vi "test.vi"() -> ()   [LabVIEW 2014]
uses:
  <vilib>/Utility/miscctls.llb/LVRectTypeDef.ctl
  <vilib>/Analysis/NI_AALBase.lvlib
panel:
  out "Numeric":i32
  out "Histogram Graph":T1(graph)
  in  "intervals":i32=10
  out "x-y":u32
  out "Image 2":u8[][](graph) caption="Image"
  out "framerate":dbl
  out "exposure":dbl
  in  "Exposure[ms]":dbl=100.0 format="%#_13g"
  out "SizeOut":T2
  in  "SizeIn":T2={"posX"=0, "posY"=0, "Width"=1024, "height"=1024}
  in  "stop":bool
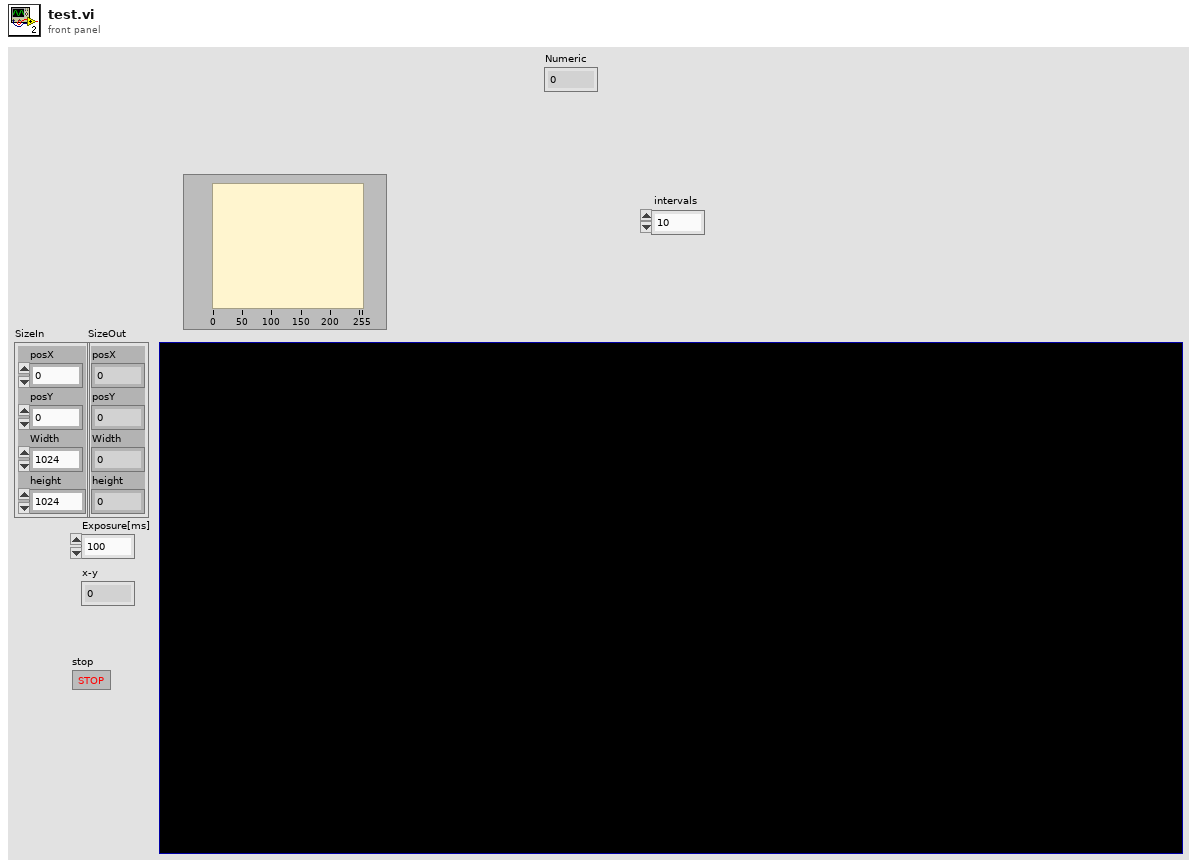
[diagram p1: front panel]
types:
  T1 = cluster{"X Values":dbl[], "Histogram: h(x)":i32[]}
  T2 = cluster{"posX":i32, "posY":i32, "Width":i32, "height":i32}
  T3 = typedef "LVRectTypeDef.ctl" = cluster{"Left":i16, "Top":i16, "Right":i16, "Bottom":i16}
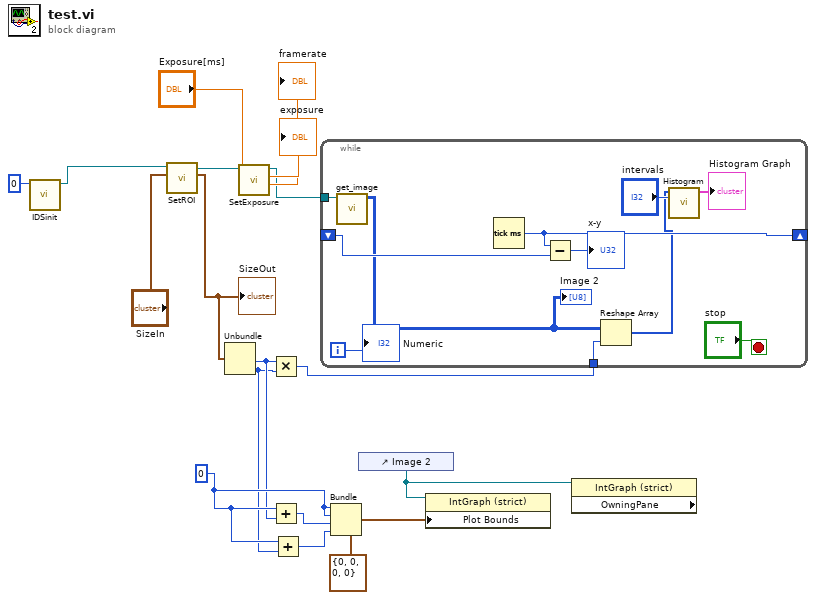
[diagram p0: block diagram]
diagram:
  w6 = i16 0 ("Left")
  n1 = call "IDSinit.vi"("Camera ID"=0) -> ("reference out"=w9:refnum<k24>)  [unwired: 6 in, 3 out]
  n2 = call "SetROI.vi"("SizeIn"="SizeIn", "reference in"=w9) -> ("SizeOut"=w11:T2, "reference out"=w16:refnum<k24>)  [unwired: 6 in, 1 out]
  "SizeOut" <- w11
  n3 = Unbundle(w11) -> ("Width"=w3:i32, "height"=w2:i32)  [unwired: 2 out]
  n4 = call "SetExposure.vi"("Exposure[ms]"="Exposure[ms]", "Reference in"=w16) -> ("framerate"=→"framerate":dbl, "exposure"=→"exposure":dbl, "reference out"=w12:refnum<k24>)  [unwired: 5 in, 1 out]
  n5 = Multiply(x=w3, y=w2) -> (x*y=w10:i32)
  n6 = Add(x=w6, y=w3) -> (x+y=w4:i32)
  n7 = Add(x=w6, y=w2) -> (x+y=w5:i32)
  n8 = while {
    tunnel: w12 -> [w28]
    shift-right: [w27] -> _
    shift-left: _ -> [w26]
    tunnel: w10 -> [w22]
    i -> [w20]
    stop <- "stop" stop-if-true
    n9 = call "get_image.vi"("reference"=w28) -> ("Array"=w19:u8[][])  [unwired: 9 in, 1 out]
    "Image 2" <- w19
    n10 = Tick Count (ms)() -> (millisecond timer value=w27:u32)
    n11 = Subtract(x=w27, y=w26) -> (x-y=→"x-y":u32)
    n12 = Reshape Array(w19, w22) -> (w21:u8[])
    n13 = call <vilib>:"Histogram.vi"("intervals"="intervals", "X"=w21) -> ("Histogram Graph"=→"Histogram Graph":T1)  [unwired: 6 in, 3 out]
    "Numeric" <- w20
  }
  n14 = Bundle(cluster=T3 {"Left"=0, "Top"=0, "Right"=0, "Bottom"=0} ("Plot Area Bounds"), "Left"=w6, "Top"=w6, "Right"=w4, "Bottom"=w5) -> (w7:T3)
  n15 = control-ref of="Image 2"() -> (w1:refnum<vi>)
  n16 = property class="IntGraph (strict)"(reference=w1, "Plot Bounds"=w7) -> ()  [unwired: 1 in, 2 out]
  n17 = property class="IntGraph (strict)" props=["OwningPane"](reference=w1) -> ()  [unwired: 1 in, 3 out]
